vi "AppleScript Global Data.vi"() -> ()   [LabVIEW 2015]
panel:
  in  "low":bool
  in  "Fire":bool
  in  "Wheel":bool
  in  "Rotate":dbl
  in  "Level":i32
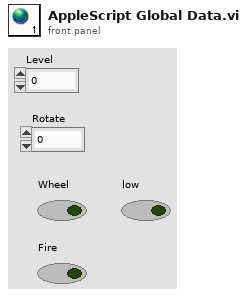
[diagram p1: front panel]
diagram:
